vi "UseMyFunction.vi"() -> ()   [LabVIEW 2020]
panel:
  out "x*y":dbl
  in  "b":dbl
  in  "c":dbl
  in  "a":dbl
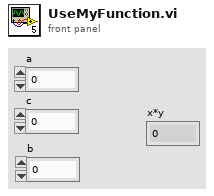
[diagram p1: front panel]
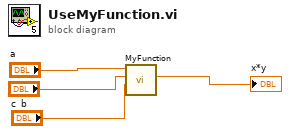
[diagram p0: block diagram]
diagram:
  n1 = call "MyFunction.vi"("c"="c", "b"="b", "a"="a") -> ("x*y"=→"x*y":dbl)  [unwired: 8 in]
